vi "NewTemplate.GetBroadcasts.vi"(11 "NewTemplate in":refnum<class "TitleBar.lvclass">) -> (2 "TemplateModule":cluster{"Broadcasts":T1, "Broadcasts":T2}, 3 "NewTemplate out":refnum<class "TitleBar.lvclass">)   [LabVIEW 2024, in "TitleBar.lvclass"]
uses:
  TitleBar.lvclass
  JQMHCore/Module/StandardBroadcasts.ctl
  JQMHCore/Shared/Died.ctl
  JQMHCore/Module/Started.ctl
  Broadcast Events--cluster.ctl
  Stopped.ctl
  JQMHCore/Module/RQMHModule.lvclass/RQMHModule.ctl
  TitleBar.lvclass/TitleBar.ctl
  JQMHCore/Module/RQMHModule.lvclass
  C:/DevOps/CORTEX/JQMH/JQMHCore/Module/RQMHModule.lvclass
  C:/DevOps/CORTEX/JQMH/ModuleTemplates/TitleBar/TitleBar.lvclass
  JQMHCore/Shared/JQMHShared.lvlib
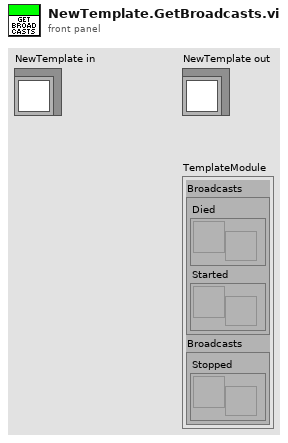
[diagram p1: front panel]
types:
  T1 = typedef "RQMHModule.lvclass/StandardBroadcasts.ctl" = cluster{"Died":refnum<user-event>, "Started":refnum<user-event>}
  T2 = typedef "TitleBar.lvclass/Broadcast Events--cluster.ctl" = cluster{"Stopped":refnum<user-event>}
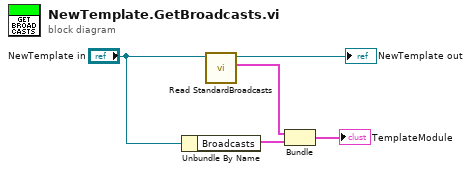
[diagram p0: block diagram]
diagram:
  n1 = Unbundle By Name("NewTemplate in") -> ("Broadcasts"=w5:T2)
  n2 = call "Read StandardBroadcasts.vi"("JQMHCore in"="NewTemplate in") -> ("Broadcasts"=w4:T1, "JQMHCore out"=→"NewTemplate out":refnum<class "TitleBar.lvclass">)  [unwired: 8 in, 1 out]
  n3 = Bundle("Broadcasts"=w4, "Broadcasts"=w5) -> (→"TemplateModule":cluster{"Broadcasts":T1, "Broadcasts":T2})  [unwired: 1 in]
